vi "Write Last Waveforms Means.vi"(8 "error in (no error)":errorcluster, 10 "Last Voltage":map{u8, dbl}(c390), 11 "Scope Base in":refnum<class "Scope Base.lvclass">) -> (0 "error out":errorcluster, 3 "Scope Base out":refnum<class "Scope Base.lvclass">)   [LabVIEW 2023]
uses:
  Scope Base.lvclass
  D:/git/HAL/Instrument/Instrument.lvclass
  D:/git/HAL/Scope Base/Scope Base.lvclass
  D:/git/HAL/Interfaces/IRead Voltage/IRead Voltage.lvclass
  D:/git/HAL/Interfaces/IScope/IScope.lvclass
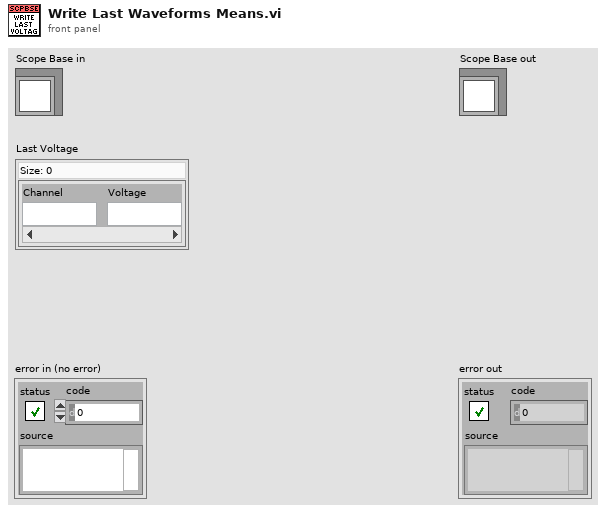
[diagram p1: front panel]
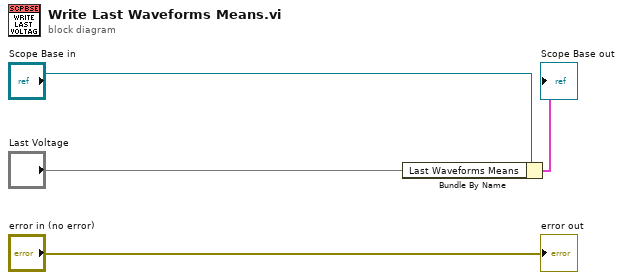
[diagram p0: block diagram]
diagram:
  n1 = Bundle By Name(cluster="Scope Base in", "Last Waveforms Means"="Last Voltage") -> (→"Scope Base out":cluster{})
  "error out" <- "error in (no error)"
